vi "Read IPS PSU Field X.vi"(8 "error in (no error)":errorcluster, 11 "Instrument.OxfordVRM in":refnum<class "Instrument.OxfordVRM.lvclass">) -> (0 "error out":errorcluster, 2 "Magnet Field (T)":dbl, 3 "Instrument.OxfordVRM out":refnum<class "Instrument.OxfordVRM.lvclass">)   [LabVIEW 2016, in "Instrument.OxfordVRM.lvclass"]
uses:
  Instrument.OxfordVRM.lvclass
  Instrument.OxfordVRM.lvclass/Instrument.OxfordVRM.ctl
  <instrlib>/Mercury iXX/Public/Libraries/Magnet/Open/Open Magnet Device.vi
  <instrlib>/Mercury iXX/Public/Libraries/Magnet/Signals/Read/Field (Read).vi
  <instrlib>/Mercury iXX/Mercury iXX.lvlib
  <instrlib>/Mercury iXX/Public/Libraries/Magnet.lvlib
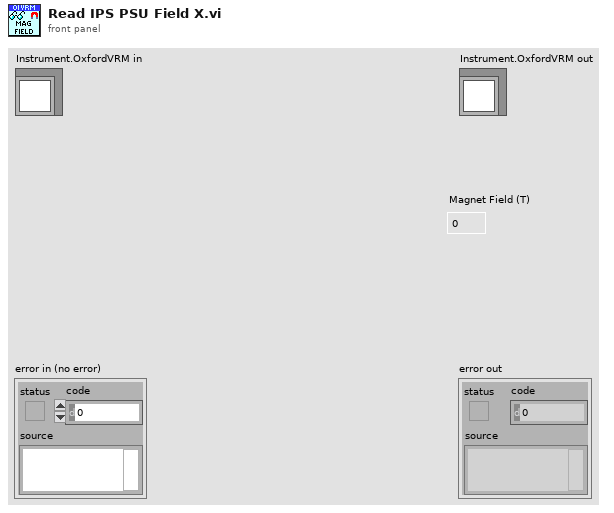
[diagram p1: front panel]
types:
  T1 = typedef "Mercury iXX.lvlib/Mercury Reference.ctl" = cluster{"Comms":refnum<visa-resource-name>, "Device ID":string[], "Comms Layer":T2, "Command":string, "Query reference":T3}
  T2 = typedef "Mercury iXX.lvlib/Comms Transport Layer.ctl" = enum16{"Ethernet TCP/IP", "USB", "ISOBus - RS-232", "GPIB"}
  T3 = typedef "Mercury iXX.lvlib/Query Dynamic Reference.ctl" = refnum<vi>
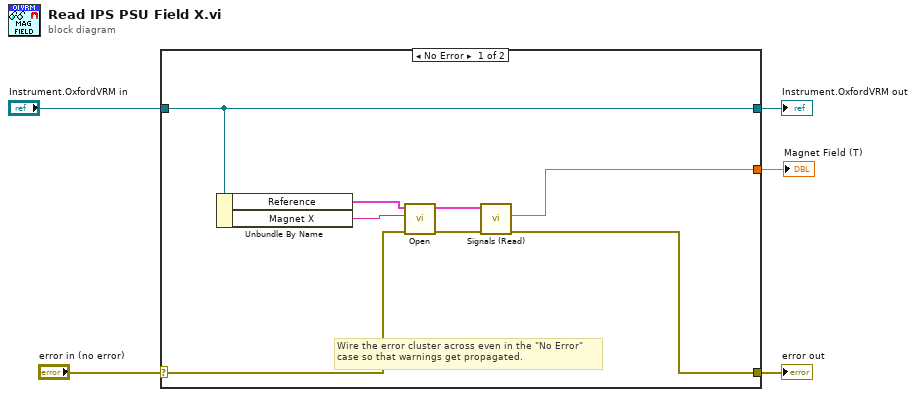
[diagram p0: block diagram]
diagram:
  n1 = case shown="No Error" "error in (no error)" {
    selector: "error in (no error)" -> [w9 w15]
    tunnel: [w8 w15] -> w4
    tunnel: [w11 w14] -> w2
    tunnel: "Instrument.OxfordVRM in" -> [w11 w14]
    tunnel: [w7 _] -> w1
    frame No Error {
      # "Wire the error cluster across even in the \"No Error\"\ncase so that warnings get propagated."
      n2 = Unbundle By Name(w11) -> ("Reference"=w6:T1, "Magnet X"=w10:string)
      n3 = call-poly <instrlib>:"Open.vi"("error in (no error)"=w9, "Device Identifier"=w10, "Mercury Reference In"=w6) -> ("error out"=w13:errorcluster, "Mercury Reference Out"=w12:T1)  [unwired: 7 out]
      n4 = call-poly <instrlib>:"Signals (Read).vi"("error in"=w13, "Mercury Reference In"=w12) -> ("error out"=w8:errorcluster, "Field"=w7:dbl)  [unwired: 1 in, 7 out]
    }
    frame Error {
    }
  }
  "error out" <- w4
  "Instrument.OxfordVRM out" <- w2
  "Magnet Field (T)" <- w1
